vi "ultimotablogin.vi"() -> ()   [LabVIEW 2018]
uses:
  controltabultimo.ctl
  controlmqultimo.ctl
panel:
  out "concatenated string":string
  out "Boolean 4":bool
  out "Boolean 3":bool
  out "Boolean 2":bool
  out "Boolean":bool
  in  "stop 3":bool
  out "coerced(x)":i32
  in  "stop 2":bool
  in  "OK Button":bool
  out "Contador de min":i32
  out "Contador de May":i32
  out "Tab Control":enum32{"Ingreso", "Usuarios", "Admin"}(tab)
  in  "Usuario Admin":string
  in  "Contraseña Admin":string
  in  "Login":bool
  in  "Usuario Ingress":string
  in  "Clave Ingress":string
  in  "Ingresar":bool
  out "Usuario a Borrar":string
  out "Clave a Borrar":string
  in  "Borrar":bool
  in  "stop":bool
  out "after substring":string
  out "match substring":string
  out "before substring":string
  out "array":string[][](array[string])
  out "element":string
  out "text":string
  out "appended path":path
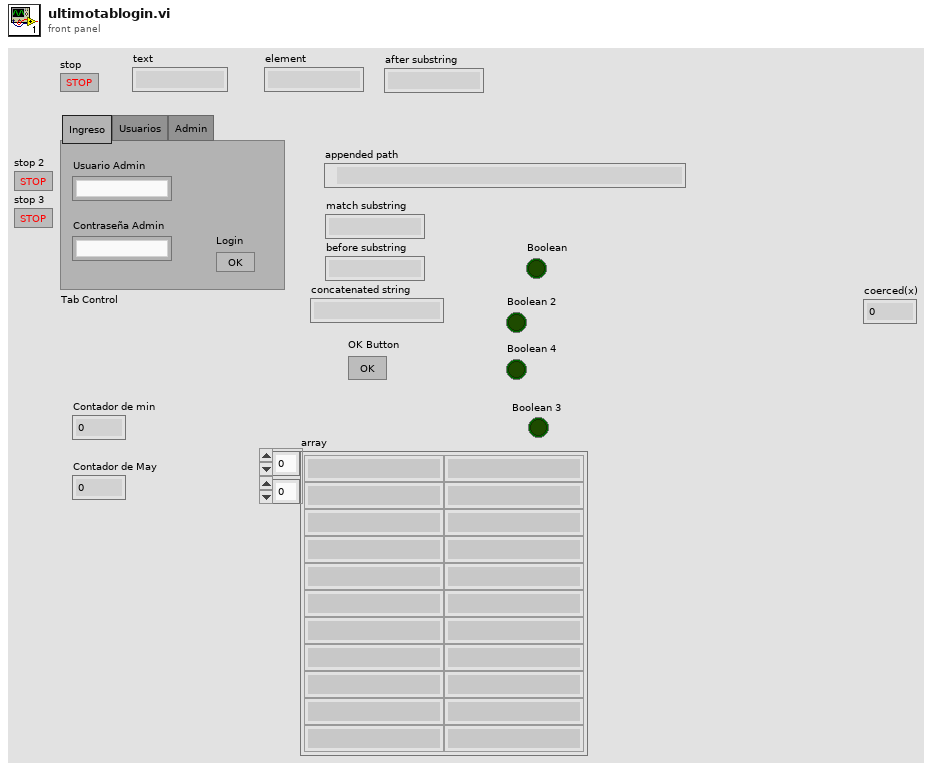
[diagram p1: front panel]
types:
  T1 = typedef "controlmqultimo.ctl" = enum16{"Control", "V.usuario/Contraseña", "V.Entre 8 y 16", "V.min y May", "Otro"}
  T2 = typedef "controltabultimo.ctl" = enum16{"Ingreso", "Usuarios", "Admin"}
  T3 = enum16{"open", "replace", "create", "open or create", "replace or create", "replace or create with confirmation"}
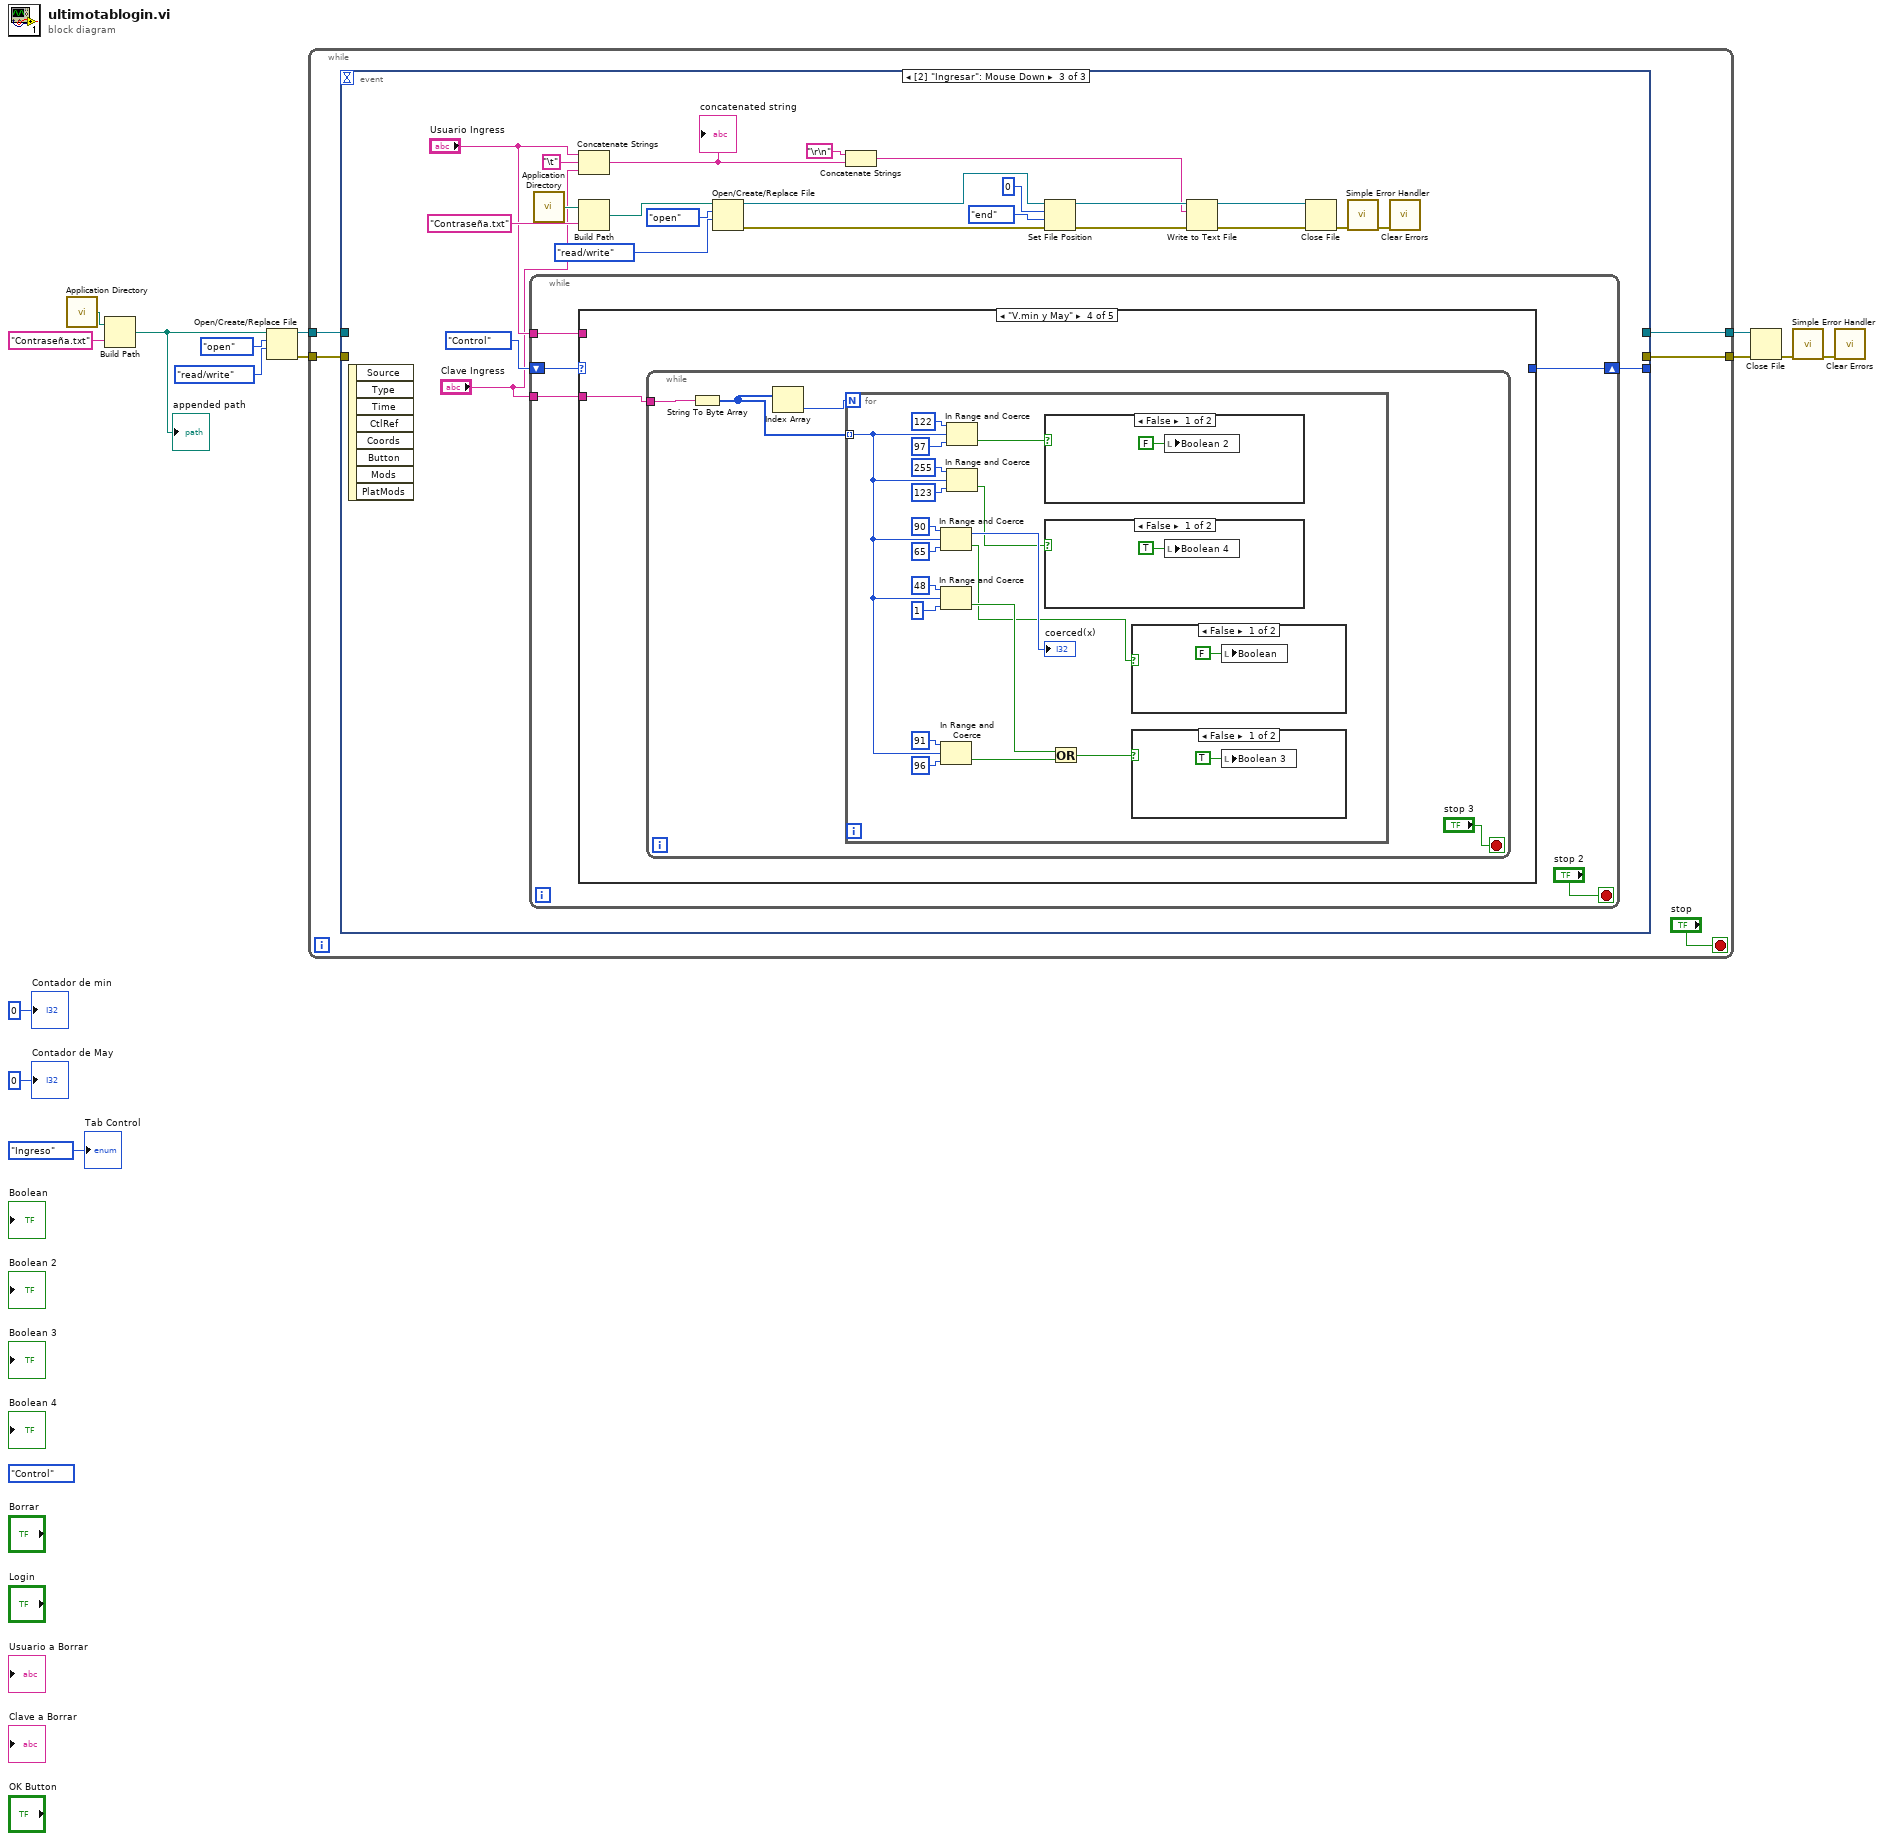
[diagram p0: block diagram]
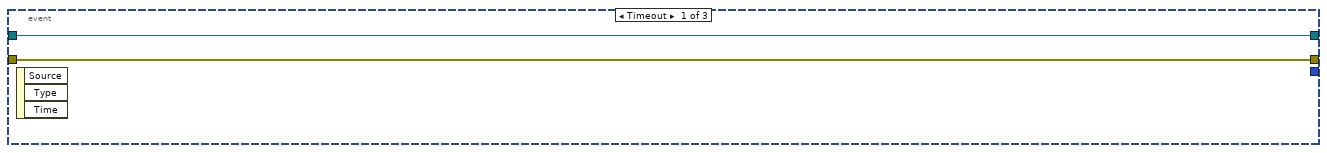
[diagram p2: hidden frame]
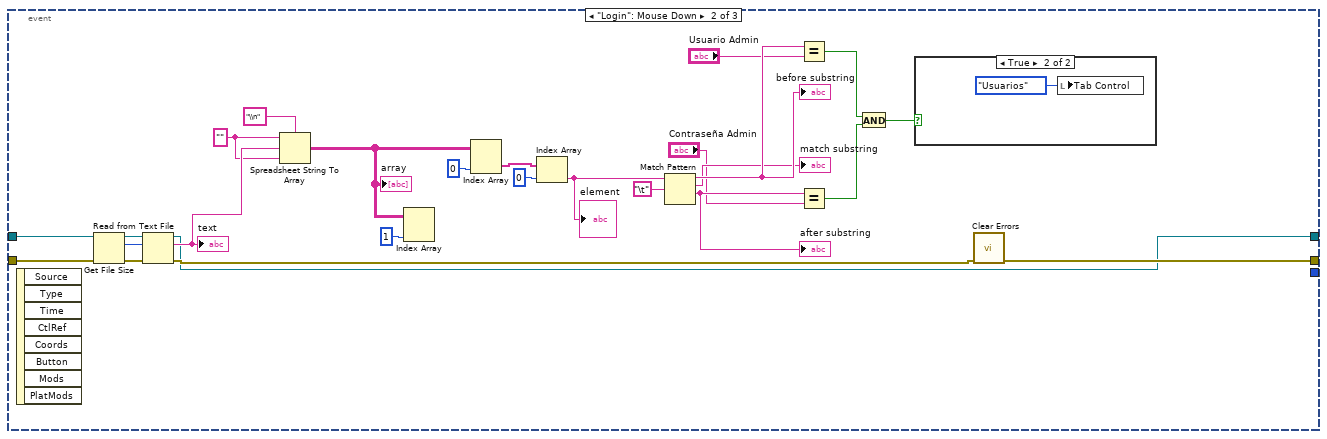
[diagram p3: hidden frame]
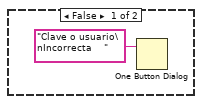
[diagram p4: hidden frame]
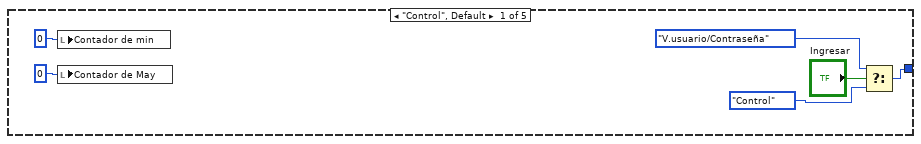
[diagram p5: hidden frame]
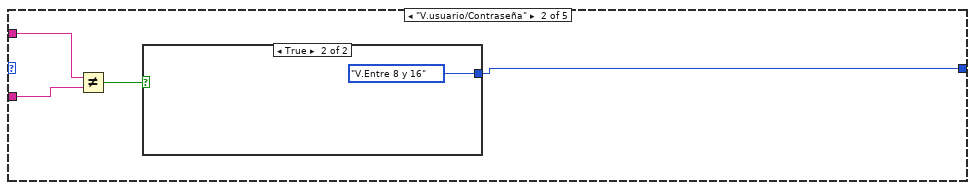
[diagram p6: hidden frame]
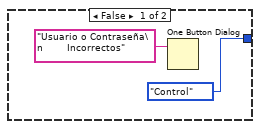
[diagram p7: hidden frame]
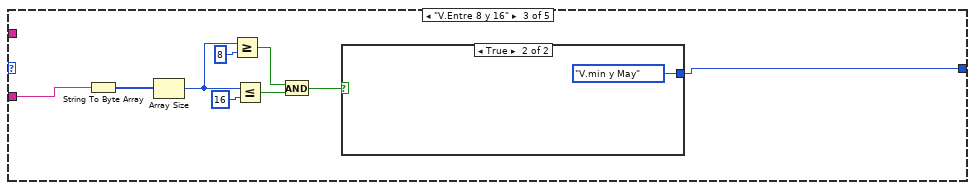
[diagram p8: hidden frame]
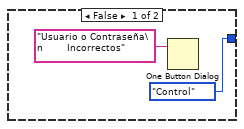
[diagram p9: hidden frame]
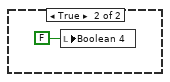
[diagram p10: hidden frame]
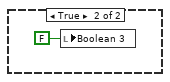
[diagram p11: hidden frame]
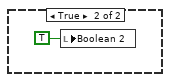
[diagram p12: hidden frame]
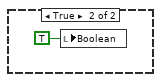
[diagram p13: hidden frame]
diagram:
  (unwired) controlmqultimo."Control"
  n1 = call <vilib>:"Application Directory.vi"() -> ("Application Directory"=w11:path)
  n2 = Build Path(base path=w11, name or relative path="Contraseña.txt") -> (appended path=w12:path)
  "appended path" <- w12
  n3 = Open/Create/Replace File(file path (use dialog)=w12, operation (0:open)=T3."open", access (0:read/write)=enum16{"read/write", "read-only", "write-only"}."read/write") -> (refnum out=w8:refnum<file>, error out=w9:errorcluster)  [unwired: 3 in, 1 out]
  n4 = while {
    tunnel: w9 -> [w19]
    tunnel: w8 -> [w18]
    tunnel: [w17] -> w5
    tunnel: [w16] -> w4
    stop <- "stop" stop-if-true
    n5 = event shown="[2] \"Ingresar\": Mouse Down" {
      selector: _ -> [_ _ _]
      dyn-events: _ -> [_ _ _]
      timeout: _ -> [_ _ _]
      tunnel: w19 -> [w21 w27 _]
      tunnel: w18 -> [w20 w28 _]
      tunnel: [w21 w24 _] -> w17
      tunnel: [w20 w23 _] -> w16
      tunnel: [_ _ w53] -> _
      event Timeout {
        n6 = event-data() -> ()  [unwired: 1 in, 3 out]
      }
      event "Login": Mouse Down {
        w29 = "" ("format string")
        n7 = event-data() -> ()  [unwired: 1 in, 8 out]
        n8 = Get File Size(file=w28, error in=w27) -> (refnum out=w47:refnum<file>, size (in bytes)=w46:i64, 0:w26:errorcluster)
        n9 = Read from Text File(file (use dialog)=w47, count=w46, error in=w26) -> (refnum out=w23:refnum<file>, text=w43:string, error out=w25:errorcluster)  [unwired: 1 in, 1 out]
        "text" <- w43
        n10 = Spreadsheet String To Array(delimiter (Tab)="\\n", format string=w29, spreadsheet string=w43, array type (2D Dbl)=w29) -> (array=w44:string[][])
        "array" <- w44
        n11 = Index Array(array=w44, index (col)=1 ("index")) -> ()  [unwired: 1 in, 1 out]
        n12 = Index Array(array=w44, index (col)=0) -> (element=w45:string[])  [unwired: 1 in]
        n13 = Index Array(array=w45, index=0) -> (element=w37:string)
        "element" <- w37
        n14 = Match Pattern(string=w37, regular expression="\t") -> (before substring=w40:string, match substring=→"match substring":string, after substring=w38:string)  [unwired: 1 in, 1 out]
        "after substring" <- w38
        "before substring" <- w40
        n15 = Equal?(x=w40, y="Usuario Admin") -> (x = y?=w41:bool)
        n16 = Equal?(x=w38, y="Contraseña Admin") -> (x = y?=w42:bool)
        n17 = And(x=w41, y=w42) -> (x .and. y?=w22:bool)
        n18 = case shown="True" w22 {
          frame False {
            n19 = One Button Dialog(message="Clave o usuario\nIncorrecta    ") -> ()  [unwired: 1 in, 1 out]
          }
          frame True {
            n20 = local write "Tab Control"(controltabultimo."Usuarios") -> ()
          }
        }
        n21 = call <vilib>:"Clear Errors.vi"("error in (no error)"=w25) -> ("error out"=w24:errorcluster)  [unwired: 5 in, 1 out]
      }
      event "Ingresar": Mouse Down {
        n22 = event-data() -> ()  [unwired: 1 in, 8 out]
        n23 = while {
          tunnel: "Usuario Ingress" -> [w76]
          shift-right: [w74] -> w53
          shift-left: controlmqultimo."Control" -> [w77]
          tunnel: "Clave Ingress" -> [w73]
          stop <- "stop 2" stop-if-true
          n24 = case shown="\"V.min y May\"" w77 {
            selector: w77 -> [_ _ _ _ w134]
            tunnel: [w80 w86 w92 _ w134] -> w74
            tunnel: w76 -> [_ w85 _ _ _]
            tunnel: w73 -> [_ w84 w91 w103 _]
            frame "Control", Default {
              n25 = local write "Contador de min"(0) -> ()
              n26 = local write "Contador de May"(0) -> ()
              n27 = Select(t=controlmqultimo."V.usuario/Contraseña", s="Ingresar", f=controlmqultimo."Control") -> (s? t:f=w80:T1)
            }
            frame "V.usuario/Contraseña" {
              n28 = Not Equal?(x=w85, y=w84) -> (x != y?=w87:bool)
              n29 = case shown="True" w87 {
                tunnel: [controlmqultimo."Control" controlmqultimo."V.Entre 8 y 16"] -> w86
                frame False {
                  n30 = One Button Dialog(message="Usuario o Contraseña\n        Incorrectos") -> ()  [unwired: 1 in, 1 out]
                }
                frame True {
                }
              }
            }
            frame "V.Entre 8 y 16" {
              n31 = String To Byte Array(string=w91) -> (unsigned byte array=w99:u8[])
              n32 = Array Size(array=w99) -> (size(s)=w98:i32)
              n33 = Greater Or Equal?(x=w98, y=8) -> (x >= y?=w95:bool)
              n34 = Less Or Equal?(x=w98, y=16) -> (x <= y?=w94:bool)
              n35 = And(x=w95, y=w94) -> (x .and. y?=w93:bool)
              n36 = case shown="True" w93 {
                tunnel: [controlmqultimo."Control" controlmqultimo."V.min y May"] -> w92
                frame False {
                  n37 = One Button Dialog(message="Usuario o Contraseña\n        Incorrectos") -> ()  [unwired: 1 in, 1 out]
                }
                frame True {
                }
              }
            }
            frame "V.min y May" {
              n38 = while {
                tunnel: w103 -> [w106]
                stop <- "stop 3" stop-if-true
                n39 = String To Byte Array(string=w106) -> (unsigned byte array=w105:u8[])
                n40 = Index Array(array=w105) -> (element=w104:u8)  [unwired: 1 in]
                n41 = for {
                  N: w104 -> [_]
                  tunnel: w105 -> [w112] mode=indexing
                  n42 = In Range and Coerce(upper limit=90, x=w112, lower limit=65) -> (coerced(x)=→"coerced(x)":i32, In Range?=w111:bool)
                  n43 = In Range and Coerce(upper limit=48, x=w112, lower limit=1) -> (In Range?=w124:bool)  [unwired: 1 out]
                  n44 = In Range and Coerce(upper limit=u8 91, x=w112, lower limit=u8 96) -> (In Range?=w125:bool)  [unwired: 1 out]
                  n45 = In Range and Coerce(upper limit=122, x=w112, lower limit=97) -> (In Range?=w110:bool)  [unwired: 1 out]
                  n46 = In Range and Coerce(upper limit=u8 255, x=w112, lower limit=u8 123) -> (In Range?=w108:bool)  [unwired: 1 out]
                  n47 = case shown="False" w110 {
                    frame False {
                      n48 = local write "Boolean 2"(FALSE) -> ()
                    }
                    frame True {
                      n49 = local write "Boolean 2"(TRUE) -> ()
                    }
                  }
                  n50 = case shown="False" w108 {
                    frame False {
                      n51 = local write "Boolean 4"(TRUE) -> ()
                    }
                    frame True {
                      n52 = local write "Boolean 4"(FALSE) -> ()
                    }
                  }
                  n53 = Or(x=w124, y=w125) -> (x .or. y?=w109:bool)
                  n54 = case shown="False" w111 {
                    frame False {
                      n55 = local write "Boolean"(FALSE) -> ()
                    }
                    frame True {
                      n56 = local write "Boolean"(TRUE) -> ()
                    }
                  }
                  n57 = case shown="False" w109 {
                    frame False {
                      n58 = local write "Boolean 3"(TRUE) -> ()
                    }
                    frame True {
                      n59 = local write "Boolean 3"(FALSE) -> ()
                    }
                  }
                }
              }
            }
            frame "Otro" {
            }
          }
        }
        n60 = call <vilib>:"Application Directory.vi"() -> ("Application Directory"=w55:path)
        n61 = Concatenate Strings "Concatenate Strings"("Usuario Ingress", "\t", "Clave Ingress") -> (w65:string)
        "concatenated string" <- w65
        n62 = Build Path(base path=w55, name or relative path="Contraseña.txt") -> (appended path=w56:path)
        n63 = Open/Create/Replace File(file path (use dialog)=w56, operation (0:open)=T3."open", access (0:read/write)=enum16{"read/write", "read-only", "write-only"}."read/write") -> (refnum out=w69:refnum<file>, error out=w70:errorcluster)  [unwired: 3 in, 1 out]
        n64 = Concatenate Strings "Concatenate Strings"("\r\n", w65) -> (w66:string)
        n65 = Set File Position(offset (in bytes) (0)=i64 0, refnum=w69, from (0:start)=enum16{"start", "end", "current"}."end", error in=w70) -> (refnum out=w71:refnum<file>, error out=w72:errorcluster)
        n66 = Write to Text File(file (use dialog)=w71, text=w66, error in=w72) -> (refnum out=w59:refnum<file>, error out=w60:errorcluster)  [unwired: 1 in, 1 out]
        n67 = Close File(refnum=w59, error in=w60) -> (error out=w58:errorcluster)  [unwired: 1 out]
        n68 = call <vilib>:"Simple Error Handler.vi"("error in (no error)"=w58) -> ("error out"=w57:errorcluster)  [unwired: 4 in, 4 out]
        n69 = call <vilib>:"Clear Errors.vi"("error in (no error)"=w57) -> ()  [unwired: 5 in, 2 out]
      }
    }
  }
  n70 = Close File(refnum=w4, error in=w5) -> (error out=w7:errorcluster)  [unwired: 1 out]
  n71 = call <vilib>:"Simple Error Handler.vi"("error in (no error)"=w7) -> ("error out"=w6:errorcluster)  [unwired: 4 in, 4 out]
  n72 = call <vilib>:"Clear Errors.vi"("error in (no error)"=w6) -> ()  [unwired: 5 in, 2 out]
  "Tab Control" <- controltabultimo."Ingreso"
  "Contador de May" <- 0 ("Contador de May")
  "Contador de min" <- 0 ("Contador de min")
